vi "GUID_Read_Default_in_editVI.vi"(8 "error in (no error)":errorcluster, 11 "GUID_Edit_path":path) -> (0 "error out":errorcluster, 1 "HostIdentifier":string, 2 "LicencePath":path, 3 ".NET GUID":string)   [LabVIEW 2018]
uses:
  <vilib>/Utility/config.llb/Read Key (String).vi
  <vilib>/Utility/config.llb/NI_LVConfig.lvlib
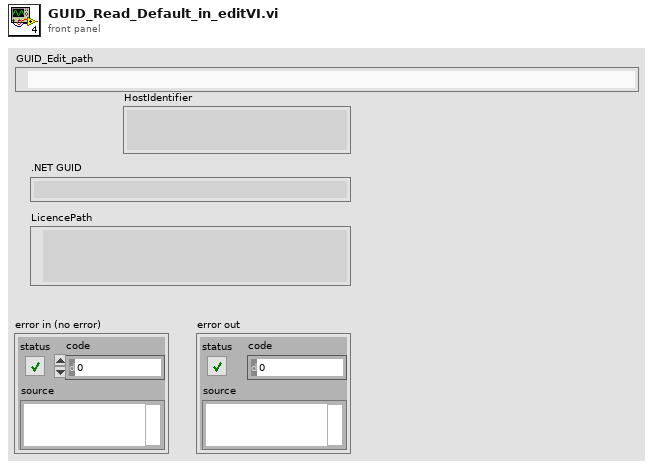
[diagram p1: front panel]
types:
  T1 = typedef "NI_LVConfig.lvlib/Config Data RefNum.ctl" = refnum<k1>
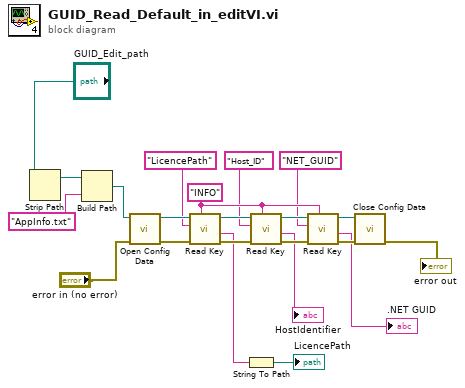
[diagram p0: block diagram]
diagram:
  w8 = "INFO" ("section")
  n1 = Strip Path(path="GUID_Edit_path") -> (stripped path=w21:path)  [unwired: 1 out]
  n2 = Build Path(base path=w21, name or relative path="AppInfo.txt") -> (appended path=w19:path)
  n3 = call <vilib>:"Open Config Data.vi"("error in (no error)"="error in (no error)", "configuration file path"=w19) -> ("error out"=w18:errorcluster, "refnum"=w17:T1)  [unwired: 7 in, 1 out]
  n4 = call-poly <vilib>:"Read Key.vi"("section"=w8, "error in (no error)"=w18, "key"="LicencePath", "refnum"=w17) -> ("error out"=w14:errorcluster, "value"=w7:string, "refnum out"=w13:T1)  [unwired: 4 in, 1 out]
  n5 = String To Path(string=w7) -> (path=→"LicencePath":path)
  n6 = call-poly <vilib>:"Read Key.vi"("section"=w8, "error in (no error)"=w14, "key"="Host_ID", "refnum"=w13) -> ("error out"=w9:errorcluster, "value"=→"HostIdentifier":string, "refnum out"=w10:T1)  [unwired: 4 in, 1 out]
  n7 = call-poly <vilib>:"Read Key.vi"("section"=w8, "error in (no error)"=w9, "key"="NET_GUID", "refnum"=w10) -> ("error out"=w12:errorcluster, "value"=→".NET GUID":string, "refnum out"=w11:T1)  [unwired: 4 in, 1 out]
  n8 = call <vilib>:"Close Config Data.vi"("error in (no error)"=w12, "refnum"=w11) -> ("error out"=→"error out":errorcluster)  [unwired: 8 in, 1 out]
